vi "paineis.vi"() -> ()   [LabVIEW 2013]
panel:
  in  "Stop Button":bool
  out "Waveform Graph":dynamicdata(graph)
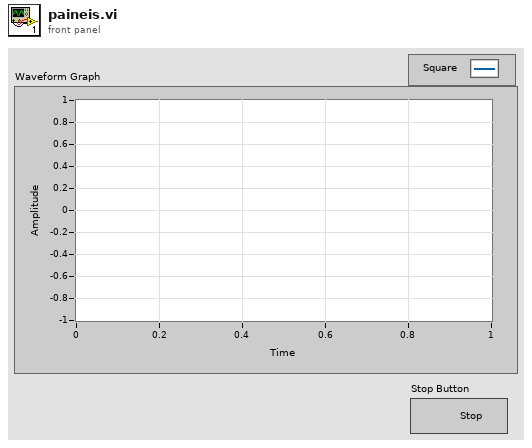
[diagram p1: front panel]
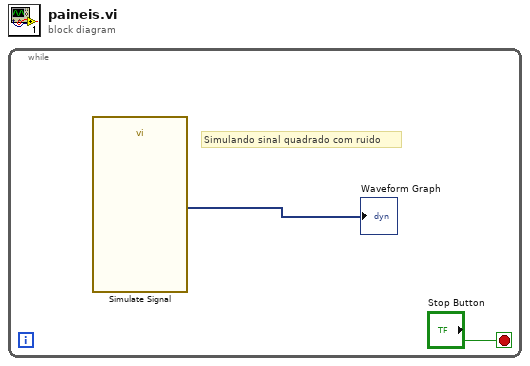
[diagram p0: block diagram]
diagram:
  n1 = while {
    stop <- "Stop Button" stop-if-true
    # "Simulando sinal quadrado com ruido"
    n2 = call "Simulate Signal"() -> ("Square"=→"Waveform Graph":dynamicdata)  [unwired: 14 in, 1 out]
  }
